vi "Move Traverse Only.vi"(7 "MoveTravBeforeTT 2":T1={"X"=-3390.0, "Y"=-113.0, "Z"=780.0, "Comment"="Anemo1", "Use Tunnel Coords?"=TRUE} caption="Move to Coords", 11 "Input Task Array":T2[](array[typedef]) {"Carrier_2 Q (l/min)" format="%#.2f"; "Row Duration (mins)" format="%#.1f"; "Row No" min=0; "Trace Gas Concentration (%)" min=0.0 format="%#_4f"; "Carrier_1 Q (l/min)" format="%#.2f"; "Tunnel Speed" format="%#.2f"; "Start X" format="%#.2f"; "Start Y" format="%#.2f"; "Start Z" format="%#.2f"; "End X" format="%#.2f"; "End Y" format="%#.2f"; "End Z" format="%#.2f"; "Averaging time (min)" min=0.0 format="%#.2f"}) -> (3 "Output Task Array":T2[](array[typedef]) {"Carrier_2 Q (l/min)" format="%#.2f"; "Row Duration (mins)" format="%#.1f"; "Row No" min=0; "Trace Gas Concentration (%)" min=0.0 format="%#_4f"; "Carrier_1 Q (l/min)" format="%#.2f"; "Tunnel Speed" format="%#.2f"; "Start X" format="%#.2f"; "Start Y" format="%#.2f"; "Start Z" format="%#.2f"; "End X" format="%#.2f"; "End Y" format="%#.2f"; "End Z" format="%#.2f"; "Averaging time (min)" min=0.0 format="%#.2f"})   [LabVIEW 2022 SP3]
uses:
  RowTemplate.ctl
  Anemometry Sub Vis/Gen Trav/Spacing.ctl
  Anemometry Sub Vis/Controls/Multi_run_mode.ctl
  MRCMDFBGlobal.vi
panel:
  # "X           Y            Z"
  # "Start"
  # "End"
  # "X           Y            Z"
  # "Start"
  # "End"
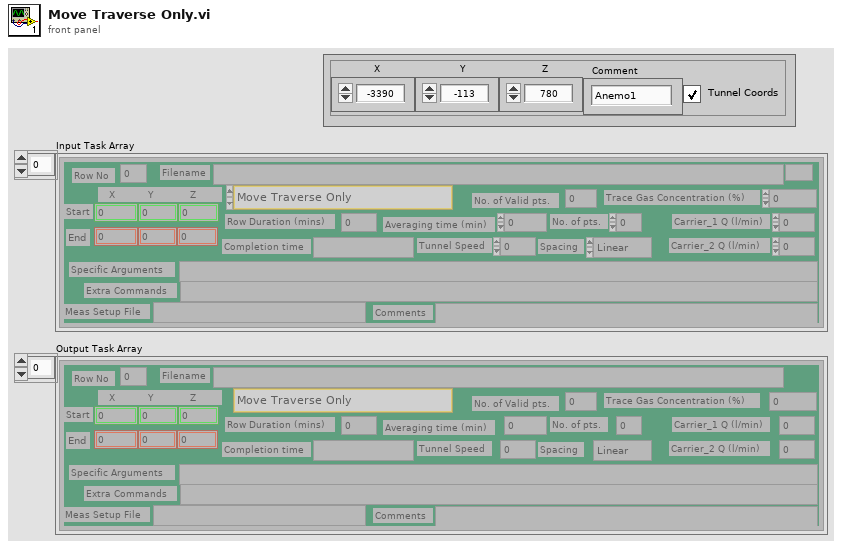
[diagram p1: front panel]
types:
  T1 = cluster{"X":dbl, "Y":dbl, "Z":dbl, "Comment":string, "Use Tunnel Coords?":bool}
  T2 = typedef "RowTemplate.ctl" = cluster{"Start X":sgl, "Start Y":sgl, "Start Z":sgl, "End X":sgl, "End Y":sgl, "End Z":sgl, "No. of pts.":i32, "Spacing":T3, "Filename":path, "Tunnel Speed":dbl, "Averaging time (min)":dbl, "Extra Commands":string, "Carrier_1 Q (l/min)":dbl, "Carrier_2 Q (l/min)":dbl, "Trace Gas Concentration (%)":dbl, "Specific Arguments":string, "Comments":string, "Row No":i32, "Row Type Selector":T4, "Completion time":string, "Row Duration (mins)":dbl, "No. of Valid pts.":i32, "Meas Setup File":string}
  T3 = typedef "Spacing.ctl" = enum16{"Linear", "Log", "Gauss", "Specified", "N/A"}
  T4 = typedef "Multi_run_mode.ctl" = enum16{"Move Traverse Only", "Set Tunnel Speed Only", "Set Source Only", "Set Measurement Conditions", "Single Measurement", "Vertical Profile", "Lateral Profile", "Longitudinal Profile", "Multi-Axis Profile", "Explore Volume", "Auto Calibrate", "Meas Fast FID Bkgnd", "Check Beam Power", "Scanning Valve Measurement", "Run VI Named:", "Set ADAM Ch", "Wait (minutes)", "Send Message", "Synchronize With:", "Fall Back to this Row", "Turn Off Row Repeating", "Traverse 3D Volume", "Blank Row", "Jump to Fall Back Row"}
  T5 = cluster{"Start X":sgl, "Start Y":sgl, "Start Z":sgl, "End X":sgl, "End Y":sgl, "End Z":sgl, "No. of pts.":i32, "Spacing":T3, "Filename":path, "Tunnel Speed":dbl, "Averaging time (min)":dbl, "Extra Commands":string, "Carrier_1 Q (l/min)":dbl, "Carrier_2 Q (l/min)":dbl, "Trace Gas Concentration (%)":dbl, "Specific Arguments":string, "Comments":string, "Row No":i32, "Row Type Selector":T4, "Completion time":string, "Row Duration (mins)":dbl, "No. of Valid pts.":i32, "Meas Setup File":string}
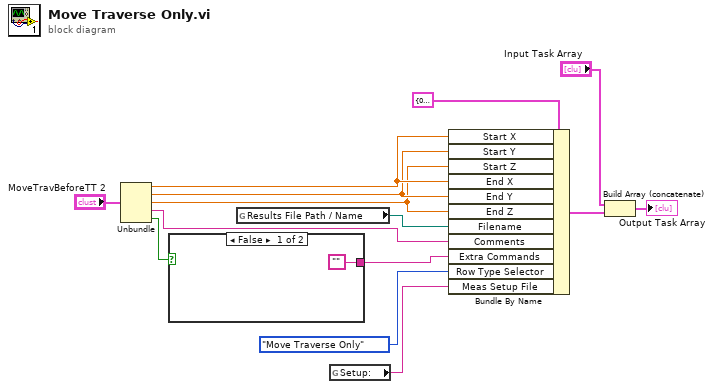
[diagram p0: block diagram]
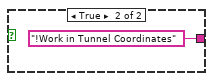
[diagram p2: hidden frame]
diagram:
  n1 = Unbundle("MoveTravBeforeTT 2") -> ("X"=w6:dbl, "Y"=w5:dbl, "Z"=w4:dbl, "Comment"=w1:string, "Use Tunnel Coords?"=w2:bool)
  n2 = case shown="False" w2 {
    tunnel: ["" "!Work in Tunnel Coordinates"] -> w7
    frame False {
    }
    frame True {
    }
  }
  n3 = global read "MRCMDFBGlobal.vi" "Results File Path / Name"() -> (w8:path)
  n4 = global read "MRCMDFBGlobal.vi" "Setup:"() -> (w9:string)
  n5 = Bundle By Name(cluster=T5 {"Start X"=0.0, "Start Y"=0.0, "Start Z"=0.0, "End X"=0.0, "End Y"=0.0, "End Z"=0.0, "No. of pts."=0, "Spacing"=enum."Linear", "Filename"=path "", "Tunnel Speed"=0.0, "Averaging time (min)"=0.0, "Extra Commands"="", "Carrier_1 Q (l/min)"=0.0, "Carrier_2 Q (l/min)"=0.0, "Trace Gas Concentration (%)"=0.0, "Specific Arguments"="", "Comments"="", "Row No"=0, "Row Type Selector"=enum."Move Traverse Only", "Completion time"="", "Row Duration (mins)"=0.0, "No. of Valid pts."=0, "Meas Setup File"=""} ("RowTemplateConst"), "Start X"=w6, "Start Y"=w5, "Start Z"=w4, "End X"=w6, "End Y"=w5, "End Z"=w4, "Filename"=w8, "Comments"=w1, "Extra Commands"=w7, "Row Type Selector"=Multi_run_mode."Move Traverse Only", "Meas Setup File"=w9) -> (w11:T5)
  n6 = Build Array (concatenate)("Input Task Array", w11) -> (→"Output Task Array":T2[])
